vi "OffsetAndBreakWaveformArray.vi"(10 "First trigger signal time":timestamp, 11 "Array":waveform(dbl)[](array[waveform])) -> (1 "Y":dbl[][](array[numeric]), 2 "dt":dbl, 3 "t":dbl)   [LabVIEW 2009]
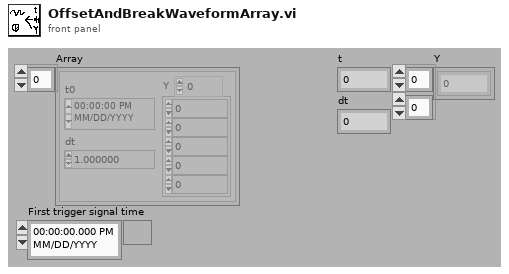
[diagram p1: front panel]
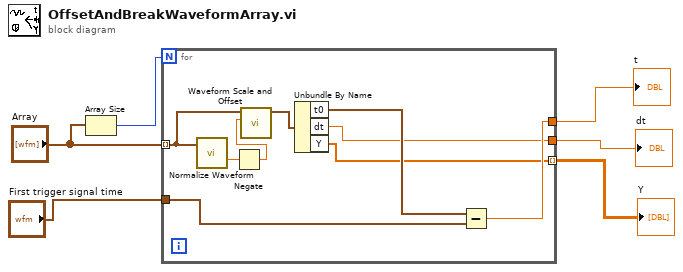
[diagram p0: block diagram]
diagram:
  n1 = Array Size(array="Array") -> (size(s)=w4:i32)
  n2 = for {
    N: w4 -> [_]
    tunnel: [w14] -> w3
    tunnel: [w13] -> w2
    tunnel: [w12] -> w1 mode=indexing
    tunnel: "Array" -> [w9] mode=indexing
    tunnel: "First trigger signal time" -> [w11]
    n3 = call <vilib>:"Normalize Waveform.vi"("waveform in"=w9) -> ("offset"=w8:dbl)  [unwired: 7 in, 3 out]
    n4 = Negate(x=w8) -> (-x=w7:dbl)
    n5 = call <vilib>:"Waveform Scale and Offset.vi"("offset"=w7, "waveform in"=w9) -> ("waveform out"=w10:waveform(dbl))  [unwired: 8 in, 1 out]
    n6 = Unbundle By Name(w10) -> ("t0"=w15:timestamp, "dt"=w13:dbl, "Y"=w12:dbl[])
    n7 = Subtract(x=w15, y=w11) -> (x-y=w14:dbl)
  }
  "t" <- w3
  "dt" <- w2
  "Y" <- w1
